vi "digital gen.vi"(8 "error in (no error)":errorcluster, 11 "PockelsCell in":refnum<class "PockelCell.lvclass">) -> (0 "error out":errorcluster, 2 "digital":variant[](array[variant]), 3 "PockelsCell out":refnum<class "PockelCell.lvclass">)   [LabVIEW 2012, in "PockelCell.lvclass"]
uses:
  PockelCell.lvclass
  PockelCell.lvclass/PockelCell.ctl
  <vilib>/Waveform/DWDTOps.llb/DWDT Boolean Array to Digital.vi
panel:
  out "analog":variant[](array[variant])
  out "settings.Duty cycle (%)":dbl(knob)=50.0 min=0.0 max=100.0 step=5.0 scale=0.0..100.0
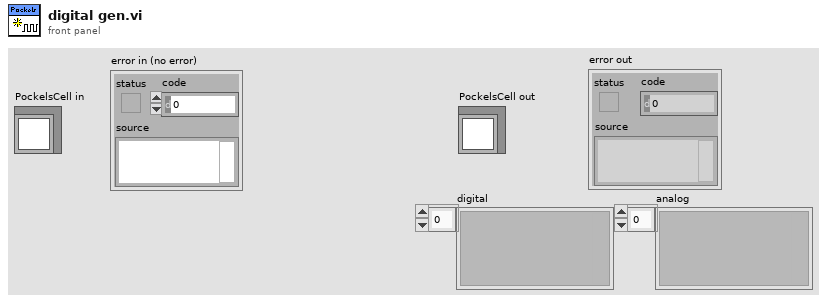
[diagram p1: front panel]
types:
  T1 = typedef "PockelCell.lvclass/laser line PC.ctl" = dbl
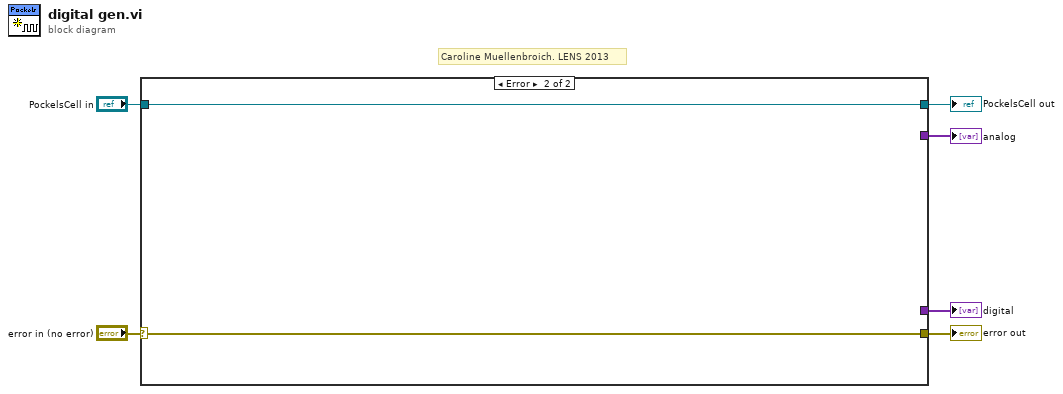
[diagram p0: block diagram]
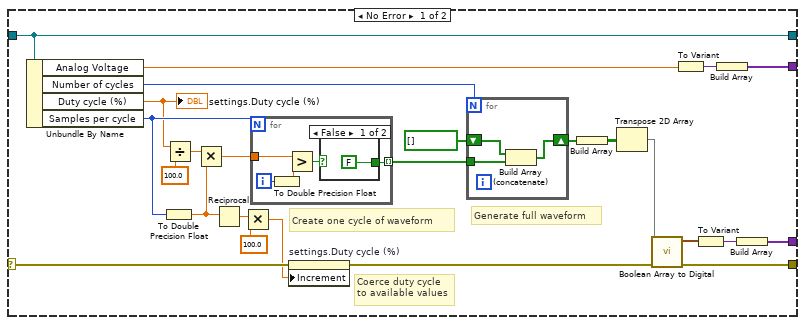
[diagram p2: hidden frame]
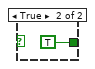
[diagram p3: hidden frame]
diagram:
  # "Caroline Muellenbroich. LENS 2013"
  n1 = case shown="Error" "error in (no error)" {
    selector: "error in (no error)" -> [w15 w43]
    tunnel: [w24 w43] -> w5
    tunnel: [w19 w42] -> w3
    tunnel: "PockelsCell in" -> [w19 w42]
    tunnel: [w10 _] -> w2
    tunnel: [w7 _] -> w1
    frame No Error {
      # "Create one cycle of waveform"
      # "Generate full waveform"
      # "Coerce duty cycle\nto available values"
      n2 = Unbundle By Name(w19) -> ("Analog Voltage"=w8:T1, "Number of cycles"=w18:i32, "Duty cycle (%)"=w16:dbl, "Samples per cycle"=w17:i32)
      "settings.Duty cycle (%)" <- w16
      n3 = To Double Precision Float(number=w17) -> (double precision float=w23:dbl)
      n4 = Divide(x=w16, y=100.0) -> (x/y=w22:dbl)
      n5 = Multiply(x=w22, y=w23) -> (x*y=w26:dbl)
      n6 = Reciprocal(x=w23) -> (1/x=w20:dbl)
      n7 = Multiply(x=w20, y=100.0) -> (x*y=w13:dbl)
      n8 = for {
        N: w17 -> [_]
        tunnel: w26 -> [w39]
        tunnel: [w37] -> w27 mode=indexing
        i -> [w36]
        n9 = To Double Precision Float(number=w36) -> (double precision float=w35:dbl)
        n10 = Greater?(x=w39, y=w35) -> (0:w38:bool)
        n11 = case shown="False" w38 {
          tunnel: [FALSE TRUE] -> w37
          frame False {
          }
          frame True {
          }
        }
      }
      n12 = property on="settings.Duty cycle (%)" class="Knob (strict)"(error in=w15, "Increment"=w13) -> (error out=w14:errorcluster)  [unwired: 1 in, 1 out]
      n13 = for {
        N: w18 -> [_]
        tunnel: w27 -> [w34]
        shift-right: [w32] -> w31
        shift-left: bool[] [] ("array") -> [w33]
        n14 = Build Array (concatenate)(w33, w34) -> (w32:bool[])
      }
      n15 = Build Array(w31) -> (w30:bool[][])
      n16 = Transpose 2D Array(2D array=w30) -> (transposed array=w29:bool[][])
      n17 = call-poly <vilib>:"Boolean Array to Digital.vi"("error in (no error)"=w14, "boolean array"=w29) -> ("error out"=w24:errorcluster, "digital waveform"=w12:digitalwaveform)  [unwired: 8 in]
      n18 = To Variant(anything=w8) -> (Variant=w9:variant)
      n19 = To Variant(anything=w12) -> (Variant=w11:variant)
      n20 = Build Array(w9) -> (w7:variant[])
      n21 = Build Array(w11) -> (w10:variant[])
    }
    frame Error {
    }
  }
  "error out" <- w5
  "PockelsCell out" <- w3
  "digital" <- w2
  "analog" <- w1
